vi "Register Plugin.vi"(6 "Version":T1, 8 "error in (no error)":errorcluster, 9 "gRPC Port":i32, 10 "Unique Name":string, 11 "Launcher in":refnum<class "Plugin Manager.lvclass">) -> (0 "error out":errorcluster, 3 "Launcher out":refnum<class "Plugin Manager.lvclass">)   [LabVIEW 2021, in "Plugin Manager.lvclass"]
uses:
  Plugin Manager.lvclass
  CIFCore/Common/Typedef/Version.ctl
  Plugin Manager.lvclass/Plugin Manager.ctl
  <vilib>/Utility/miscctls.llb/LVMapReplaceAction.ctl
  CIFCore/Common/Typedef/Errors.ctl
  CIFCore/Common/Utilities/Append Error Location.vi
  CIFCore/Common/CIFCoreCommon.lvlib
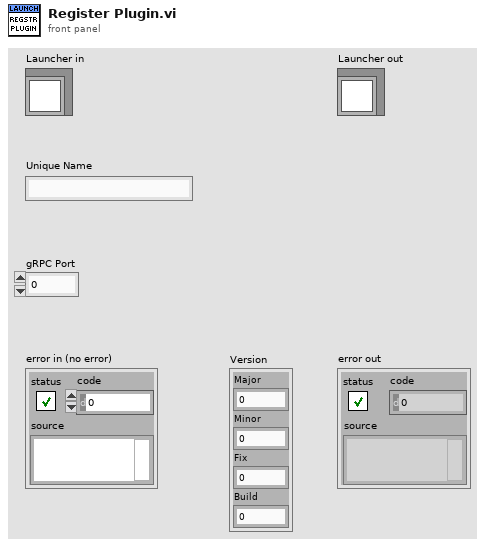
[diagram p1: front panel]
types:
  T1 = typedef "CIFCoreCommon.lvlib/Version.ctl" = cluster{"Major":i32, "Minor":i32, "Fix":i32, "Build":i32}
  T2 = typedef "LVMapReplaceAction.ctl" = enum32{"Modify Entry only if found", "Add or Modify Entry", "Delete Entry"}
  T3 = typedef "CIFCoreCommon.lvlib/Errors.ctl" = enum16{"Invalid Clock ID", "Long Sleep", "gRPC Server Not Found", "Config Parse", "Timestamp Wrap", "Delayed Execution", "Duplicate Channel", "Missing Channel", "Incorrect Type", "Flatten Error", "Unflatten Data", "Unique Name", "Plugin Not Found"}
  T4 = typedef "Plugin Manager.lvclass/Plugin Management Data.ctl" = cluster{"vi reference":refnum<vi>, "Plugin Type":string, "Unique Name":string, "Load Timestamp":u64, "gRPC Port":i32, "Version":T1}
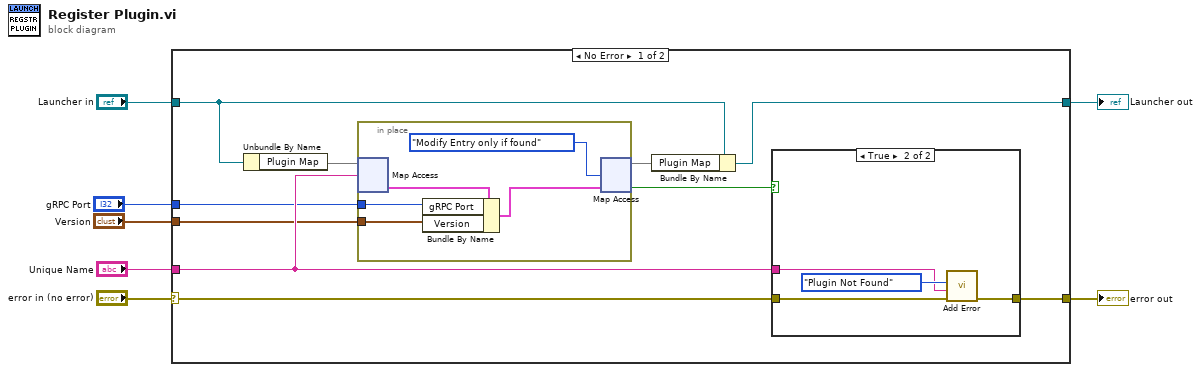
[diagram p0: block diagram]
diagram:
  n1 = case shown="No Error" "error in (no error)" {
    selector: "error in (no error)" -> [w17 w29]
    tunnel: [w16 w29] -> w6
    tunnel: [w8 w28] -> w4
    tunnel: "Launcher in" -> [w11 w28]
    tunnel: "Unique Name" -> [w14 _]
    tunnel: "Version" -> [w13 _]
    tunnel: "gRPC Port" -> [w12 _]
    frame No Error {
      n2 = Unbundle By Name(w11) -> ("Plugin Map"=w15:map{string, T4})
      n3 = in-place {
        in-place-border: w13 -> [w20]
        in-place-border: w12 -> [w19]
        n4 = in-place-map #1(w15, w14) -> (w21:T4)  [unwired: 1 in, 1 out]
        n5 = Bundle By Name(cluster=w21, "gRPC Port"=w19, "Version"=w20) -> (w18:T4)
        n6 = in-place-map #1(w18, LVMapReplaceAction."Modify Entry only if found" ("action")) -> (w10:map{string, T4}, w9:bool)  [unwired: 1 out]
      }
      n7 = Bundle By Name(cluster=w11, "Plugin Map"=w10) -> (w8:refnum<class "Plugin Manager.lvclass">)
      n8 = case shown="True" w9 {
        tunnel: w17 -> [w23 w27]
        tunnel: [w23 w24] -> w16
        tunnel: w14 -> [_ w25]
        frame False {
        }
        frame True {
          n9 = call "Add Error.vi"("error in (no error)"=w27, "String to Append"=w25, "Error"=Errors."Plugin Not Found") -> ("error out"=w24:errorcluster)  [unwired: 8 in]
        }
      }
    }
    frame Error {
    }
  }
  "error out" <- w6
  "Launcher out" <- w4
